vi "Random.vi"(6 "Write?":bool, 9 "lower bound(ms)":dbl, 10 "upper bound(ms)":dbl, 11 "ExecuteTime(s)":dbl=5.0 caption="Execute:" min=1.0 format="%#.3gs") -> (2 "Time Target (s)":dbl caption="数字")   [LabVIEW 2020]
uses:
  <vilib>/numeric/Random Number (Range) DBL.vi
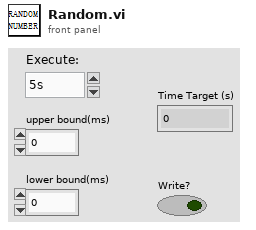
[diagram p1: front panel]
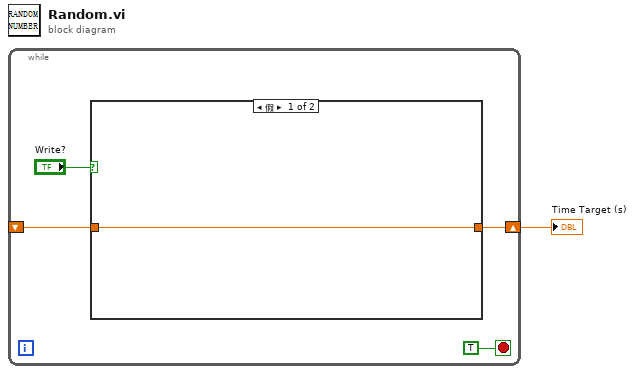
[diagram p0: block diagram]
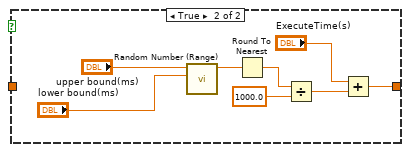
[diagram p2: hidden frame]
diagram:
  n1 = while {
    shift-right: [w5] -> w1
    shift-left: _ -> [w4]
    stop <- TRUE stop-if-true
    n2 = case shown="假" "Write?" {
      tunnel: [w6 w7] -> w5
      tunnel: w4 -> [w6 _]
      frame False {
      }
      frame True {
        n3 = call-poly <vilib>:"Random Number (Range).vi"("lower bound (0)"="lower bound(ms)", "upper bound (100)"="upper bound(ms)") -> ("number"=w11:dbl)  [unwired: 9 in]
        n4 = Round To Nearest(number=w11) -> (nearest integer value=w10:dbl)
        n5 = Divide(x=w10, y=1000.0) -> (x/y=w9:dbl)
        n6 = Add(x="ExecuteTime(s)", y=w9) -> (x+y=w7:dbl)
      }
    }
  }
  "Time Target (s)" <- w1
